vi "3Act Helper - NormalizePWMRatio.vi"(9 "Ratio In":dbl, 10 "Maximum ratio":dbl=1.0 format="%#_13g") -> (2 "Normalized Ratio":dbl)   [LabVIEW 2013]
doc: "Takes in a 0-1 ratio of high PWM signal to total PWM cycle length."
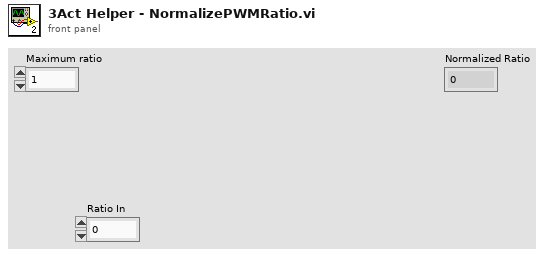
[diagram p1: front panel]
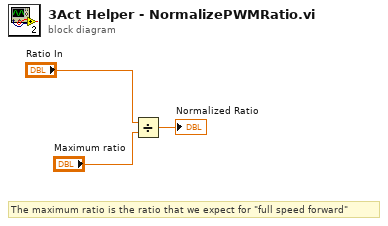
[diagram p0: block diagram]
diagram:
  # "The maximum ratio is the ratio that we expect for \"full speed forward\""
  n1 = Divide(x="Ratio In", y="Maximum ratio") -> (x/y=→"Normalized Ratio":dbl)
